vi "Auto_Routine_RightTwoPieceThen2CenterTRAJ.vi"   [LabVIEW 2023]
uses:
  Shoulder/ShoulderGetSetpointEnum.ctl
  Trajectory/TrajectoryGlobals.vi
  <vilib>/Rock Robotics/WPI/ThirdParty/JAS_Junk/TrajLib/Trajectory_Library.lvlib
types:
  T1 = typedef "ShoulderGetSetpointEnum.ctl" = enum16{"ArmFloorPickup", "ArmAmpDeposit", "ArmSpeakerShoot", "ArmStartPosition", "ArmRestPosition", "ArmSourceIntake", "ArmAwayShoot"}
  T2 = typedef "Trajectory_Library.lvlib/TRAJECTORY.ctl" = cluster{"TotalTImeSecs":dbl, "States":T3[]}
  T3 = typedef "Trajectory_Library.lvlib/TRAJ_STATE.ctl" = cluster{"TimeSeconds":dbl, "Velocity":dbl, "Acceleration":dbl, "POSE":T4, "Curvature":dbl}
  T4 = typedef "Trajectory_Library.lvlib/POSE2D.ctl" = cluster{"TRANSLATION":T5, "ROTATION":T6}
  T5 = typedef "Trajectory_Library.lvlib/TRANSLATION2D.ctl" = cluster{"X":dbl, "Y":dbl}
  T6 = typedef "Trajectory_Library.lvlib/ROTATION2D.ctl" = cluster{"VALUE":dbl, "COS":dbl, "SIN":dbl}
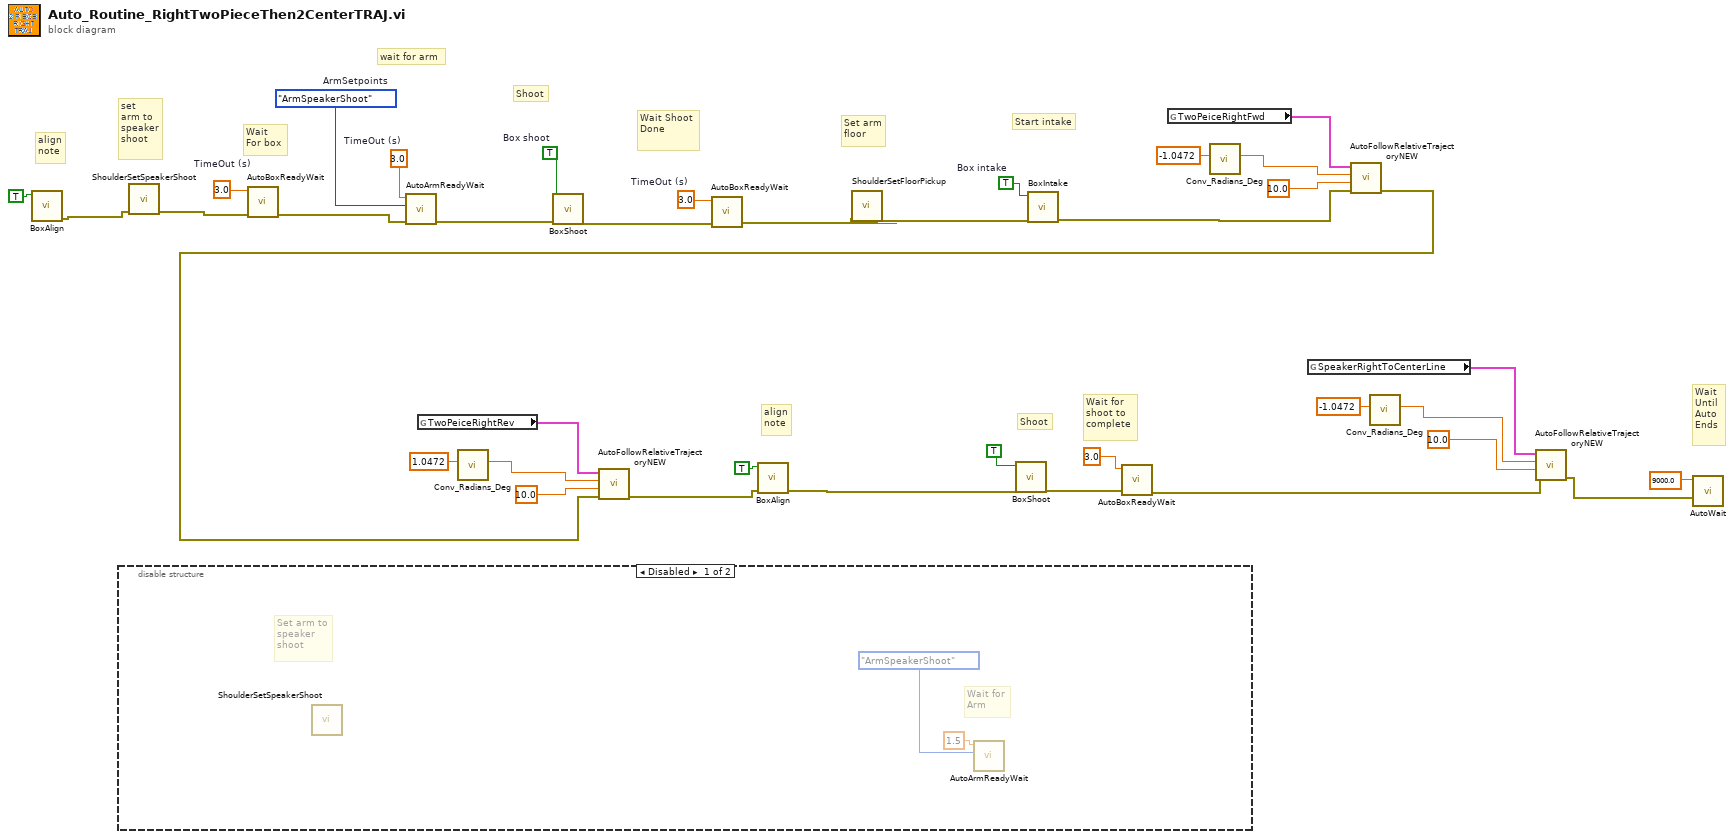
[diagram p0: block diagram]
diagram:
  w27 = 3.0  # TimeOut (s)
  w37 = TRUE  # Box intake
  w36 = TRUE  # Box shoot
  w35 = ShoulderGetSetpointEnum."ArmSpeakerShoot"  # ArmSetpoints
  w34 = 3.0  # TimeOut (s)
  w30 = 3.0  # TimeOut (s)
  # "align\nnote"
  # "Wait\nUntil\nAuto \nEnds"
  # "Wait for\nshoot to\ncomplete"
  # "Shoot"
  # "Start intake"
  # "Set arm\nfloor"
  # "Wait Shoot\nDone"
  # "Shoot"
  # "Wait\nFor box"
  # "set \narm to\nspeaker\nshoot"
  # "align\nnote"
  # "wait for arm"
  n1 = call "BoxAlign.vi"("box align"=TRUE) -> ("error out"=w28:errorcluster)  [unwired: 10 in]
  n2 = disable-structure shown="Disabled" {
    frame Disabled {
      # "Wait for\nArm"
      # "Set arm to\nspeaker \nshoot"
      n3 = call "ShoulderSetSpeakerShoot.vi"() -> ()  [unwired: 11 in, 1 out]
      n4 = call "AutoArmReadyWait.vi"("ArmSetpoints"=ShoulderGetSetpointEnum."ArmSpeakerShoot", "TimeOut (s)"=1.5) -> ("error in (no error)"=w38:errorcluster)  [unwired: 8 in, 1 out]
    }
    frame Enabled {
    }
  }
  n5 = call "ShoulderSetSpeakerShoot.vi"("error in (no error)"=w28) -> ("error out"=w26:errorcluster)  [unwired: 10 in]
  n6 = call "AutoBoxReadyWait.vi"("error in (no error)"=w26, "TimeOut (s)"=w27) -> ("error out"=w25:errorcluster)  [unwired: 9 in]
  n7 = call "AutoArmReadyWait.vi"("error in (no error)"=w25, "ArmSetpoints"=w35, "TimeOut (s)"=w34) -> ("error out"=w31:errorcluster)  [unwired: 8 in]
  n8 = global read "TrajectoryGlobals.vi" "TwoPeiceRightRev"() -> (w14:T2)
  n9 = call <vilib>:"Conv_Radians_Deg.vi"("Radians"=1.0472) -> ("Degrees"=w12:dbl)  [unwired: 10 in]
  n10 = call "BoxShoot.vi"("error in (no error)"=w31, "Box shoot"=w36) -> ("error out"=w32:errorcluster)  [unwired: 9 in]
  n11 = call "AutoBoxReadyWait.vi"("error in (no error)"=w32, "TimeOut (s)"=w30) -> ("error out"=w24:errorcluster)  [unwired: 9 in]
  n12 = call "ShoulderSetFloorPickup.vi"("error in (no error)"=w24) -> ("error out"=w33:errorcluster)  [unwired: 10 in]
  n13 = call "BoxIntake.vi"("error in (no error)"=w33, "Box intake"=w37) -> ("error out"=w23:errorcluster)  [unwired: 9 in]
  n14 = global read "TrajectoryGlobals.vi" "TwoPeiceRightFwd"() -> (w22:T2)
  n15 = call <vilib>:"Conv_Radians_Deg.vi"("Radians"=-1.0472) -> ("Degrees"=w20:dbl)  [unwired: 10 in]
  n16 = global read "TrajectoryGlobals.vi" "SpeakerRightToCenterLine"() -> (w8:T2)
  n17 = call "AutoFollowRelativeTrajectoryNEW.vi"("error in (no error)"=w23, "TimeOut (s)"=10.0, "End Orientation"=w20, "Trajectory"=w22) -> ("error out"=w2:errorcluster)  [unwired: 7 in]
  n18 = call "AutoFollowRelativeTrajectoryNEW.vi"("error in (no error)"=w2, "TimeOut (s)"=10.0, "End Orientation"=w12, "Trajectory"=w14) -> ("error out"=w9:errorcluster)  [unwired: 7 in]
  n19 = call "BoxAlign.vi"("error in (no error)"=w9, "box align"=TRUE) -> ("error out"=w1:errorcluster)  [unwired: 9 in]
  n20 = call "BoxShoot.vi"("error in (no error)"=w1, "Box shoot"=TRUE) -> ("error out"=w17:errorcluster)  [unwired: 9 in]
  n21 = call "AutoBoxReadyWait.vi"("error in (no error)"=w17, "TimeOut (s)"=3.0) -> ("error out"=w4:errorcluster)  [unwired: 9 in]
  n22 = call <vilib>:"Conv_Radians_Deg.vi"("Radians"=-1.0472) -> ("Degrees"=w6:dbl)  [unwired: 10 in]
  n23 = call "AutoFollowRelativeTrajectoryNEW.vi"("error in (no error)"=w4, "TimeOut (s)"=10.0, "End Orientation"=w6, "Trajectory"=w8) -> ("error out"=w3:errorcluster)  [unwired: 7 in]
  n24 = call "AutoWait.vi"("error in (no error)"=w3, "TimeOut (s)"=9000.0) -> ()  [unwired: 9 in, 1 out]
